vi "GUI_picoscope.vi"() -> ()   [LabVIEW 2020]
uses:
  Device Drivers/ScopeAnalysis/SubVis/method_TypDef.ctl
  Device Drivers/ScopeAnalysis/SubVis/channels_TypDef.ctl
  Shared/GUI_Template/GUI_master/tcp new data cluster.ctl
  General-Controler/firstCall_TypDef.ctl
panel:
  in  "TimeAxis.Max Sample Points::1":T1(ring)=enum."5k" caption="Max record length"
  in  "Trigger.Source::1":u16(ring) caption="Source" items=["Channel 1", "Channel 2", "Channel 3", "Channel 4", "External", "Power Line"]
  in  "Analysis":T4={"Channel::1"=enum."Analysis1", "Calculations.Method::1"=enum."trigger", "Measurements::1"=-5e-07, "Calculations.Linked::1"=enum."na", "Calculations.Additional::1"=0.0} {"Calculations.Additional::1" min=0.0 max=0.0; "Measurements::1" min=0.0 max=0.0}
  in  "TimeAxis.Time base::1":dbl=500000000.0 caption="Time interval" min=0.0 max=0.0 step=1000000.0 format="%.0p"
  in  "Trigger.mode::1":u16(ring) caption="Mode" items=["Auto", "Normal", "Single", "Single auto trigger"]
  in  "Trigger.Level::1":dbl=0.5 caption="Level" min=0.0 max=0.0 format="%#_6p"
  in  "Trigger.Slope::1":u16(ring) caption="Slope" items=["Rising", "Falling"]
  in  "autoscale::1":bool caption="auto\nscale"
  in  "LocalSavingPath::1":path
  in  "save::1":bool=TRUE caption="save"
  in  "Select device":string(combo)="StagingPXIFast1"
  in  "Refresh Button":bool
  out "device status::1":string="Initialized" caption="Device status"
  in  "stop":bool=TRUE
  out "GUIdevice 1":string="StagingPXIFast1"
  in  "Waveform cluster":T5={"Channel::1"=enum."Channel0", "coupling::1"=1, "Verticaloffset::1"=0.0, "Chenabled::1"=1, "verticalrange::1"=0.1, "Names::1"="", "scopeTraceGUI::1"=[{"t0"=timestamp(-4.999999999588667e-07 s since 1904-01-01), "dt"=2e-09, "Y"=array[1000 elements]}, {"t0"=timestamp(-4.999999999588667e-07 s since 1904-01-01), "dt"=2e-09, "Y"=array[1000 elements]}]} {"verticalrange::1" min=0.0001 max=30.0 format="%_4f"; "Chenabled::1" items=["off", "on"]; "Verticaloffset::1" min=-5.0 max=5.0; "coupling::1" items=["AC", "DC"]}
  # "TRIGGER"
  # "HORIZONTAL"
  # "ANALYSIS"
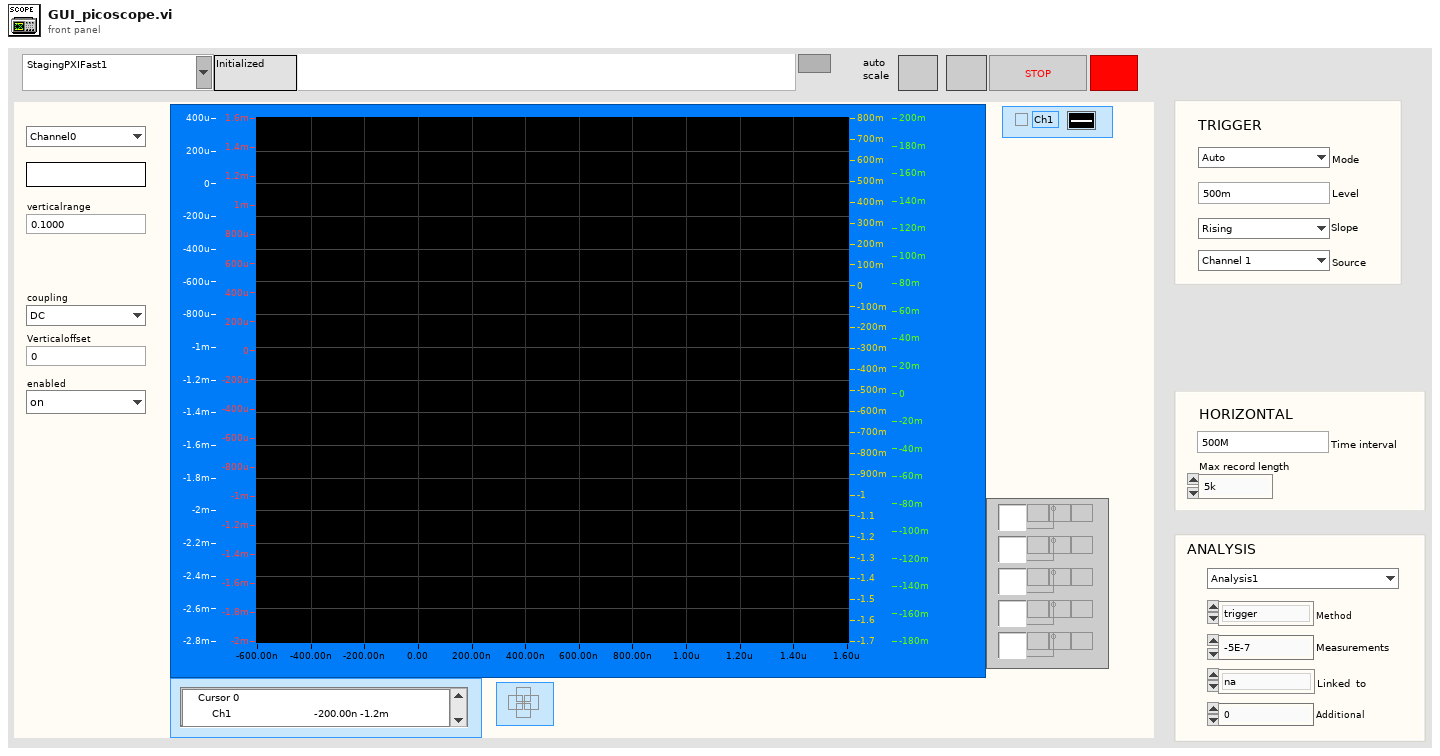
[diagram p1: front panel]
types:
  T1 = enum16{"50", "100", "250", "500", "1000", "2500", "5k", "10k", "25k", "50k", "100k", "250k", "500k", "1M", "2M", "2.5M", "5M", "10M", "25M", "50M", "100M"}
  T2 = typedef "method_TypDef.ctl" = enum16{"n/a", "max", "min", "energy", "trigger", "maxtime", "mintime"}
  T3 = typedef "channels_TypDef.ctl" = enum16{"na", "StagingPXIFast1 scopeTrace.Channel0", "StagingPXIFast1 scopeTrace.Channel1", "StagingPXIFast2 scopeTrace.Channel0", "StagingPXIFast2 scopeTrace.Channel1", "StagingPXISlow scopeTrace.Channel0", "StagingPXISlow scopeTrace.Channel1", "StagingPXISlow scopeTrace.Channel2", "StagingPXISlow scopeTrace.Channel3", "StagingPXISlow scopeTrace.Channel4", "StagingPXISlow scopeTrace.Channel5", "StagingPXISlow scopeTrace.Channel6", "StagingPXISlow scopeTrace.Channel7"}
  T4 = cluster{"Channel::1":enum16{"Analysis1", "Analysis2", "Analysis3", "Analysis4", "Analysis5", "Analysis6", "Analysis7", "Analysis8", "Analysis9"}, "Calculations.Method::1":T2, "Measurements::1":dbl, "Calculations.Linked::1":T3, "Calculations.Additional::1":dbl}
  T5 = cluster{"Channel::1":enum16{"Channel0", "Channel1", "Channel2", "Channel3", "Channel4", "Channel5", "Channel6", "Channel7"}, "coupling::1":u16, "Verticaloffset::1":dbl, "Chenabled::1":u16, "verticalrange::1":dbl, "Names::1":string, "scopeTraceGUI::1":waveform(dbl)[]}
  T6 = typedef "tcp new data cluster.ctl" = cluster{"EventEnum":enum16{"new data", "connection status update"}, "Device name":string}
  T7 = typedef "firstCall_TypDef.ctl" = enum16{"reset", "read"}
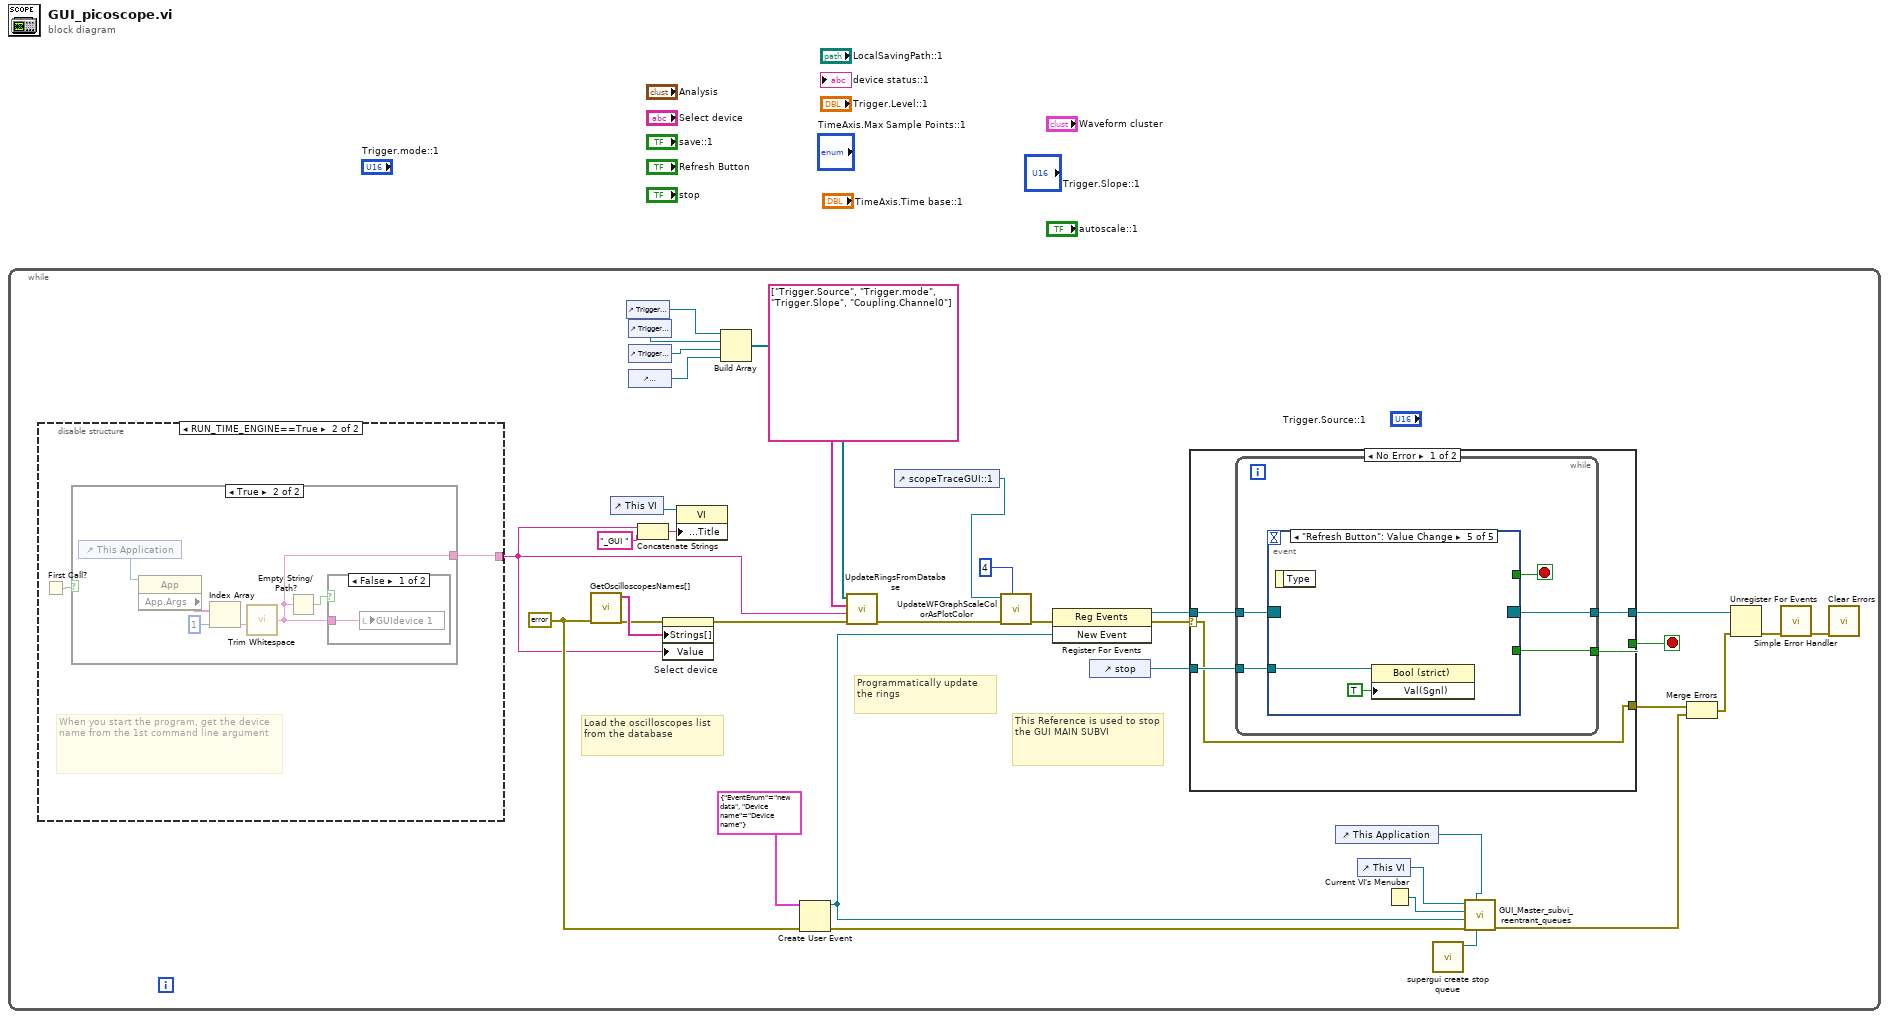
[diagram p0: block diagram]
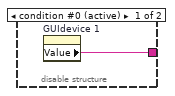
[diagram p2: hidden frame]
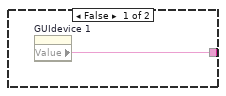
[diagram p3: hidden frame]
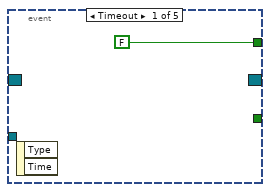
[diagram p5: hidden frame]
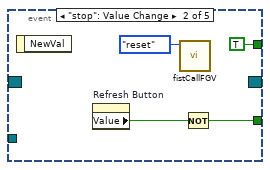
[diagram p6: hidden frame]
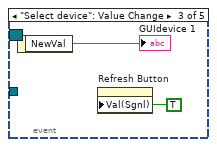
[diagram p7: hidden frame]
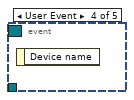
[diagram p8: hidden frame]
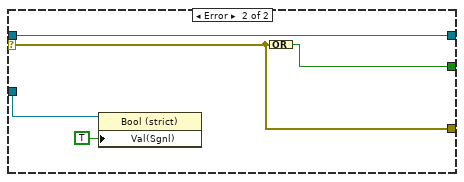
[diagram p9: hidden frame]
diagram:
  n1 = while {
    stop <- w33 stop-if-true
    w7 = errorcluster {"status"=FALSE, "code"=0, "source"=""} ("error in (no error)")
    # "Programmatically update the rings"
    # "Load the oscilloscopes list from the database"
    # "This Reference is used to stop the GUI MAIN SUBVI"
    n2 = disable-structure shown="RUN_TIME_ENGINE==True" {
      disable-tunnel: [w36 w37] -> w1
      frame condition #0 (active) {
        n3 = property on="GUIdevice 1" class="Str"() -> ("Value"=w36:string)  [unwired: 2 in, 2 out]
      }
      frame condition #1 {
        # "When you start the program, get the device name from the 1st command line argument"
        n4 = First Call?() -> (First Call?: T/F=w38:bool)
        n5 = case shown="True" w38 {
          tunnel: [w39 w40] -> w37
          frame False {
            n6 = property on="GUIdevice 1" class="Str"() -> ("Value"=w39:string)  [unwired: 2 in, 2 out]
          }
          frame True {
            n7 = control-ref of="This Application"() -> (w42:refnum<vi>)
            n8 = property class="App"(reference=w42) -> ("App.Args"=w43:string[])  [unwired: 1 in, 2 out]
            n9 = Index Array(array=w43, index=1) -> (element=w44:string)
            n10 = call <vilib>:"Trim Whitespace.vi"("string"=w44) -> ("trimmed string"=w40:string)  [unwired: 1 in]
            n11 = Empty String/Path?(string/path=w40) -> (empty?=w45:bool)
            n12 = case shown="False" w45 {
              tunnel: w40 -> [w46 _]
              frame False {
                n13 = local write "GUIdevice 1"(w46) -> ()
              }
              frame True {
              }
            }
          }
        }
      }
    }
    n14 = call "GetOscilloscopesNames[].vi"("error in (no error)"=w7) -> ("error IO"=w24:errorcluster, "OscilloscopesNames[]"=w25:string[])  [unwired: 9 in]
    n15 = control-ref of="This VI"() -> (w4:refnum<vi>)
    n16 = control-ref of="Trigger.Source::1"() -> (w6:refnum<vi>)
    n17 = control-ref of="Trigger.mode::1"() -> (w22:refnum<vi>)
    n18 = control-ref of="Trigger.Slope::1"() -> (w21:refnum<vi>)
    n19 = control-ref of="Coupling::1"() -> (w20:refnum<vi>)
    n20 = Concatenate Strings(w1, "_GUI ") -> (w3:string)
    n21 = property on="Select device" class="CmbBox"(error in=w24, "Strings[]"=w25, "Value"=w1) -> (error out=w23:errorcluster)  [unwired: 1 in, 1 out]
    n22 = property class="VI"(reference=w4, "Front Panel.Title"=w3) -> ()  [unwired: 1 in, 2 out]
    n23 = Build Array(w6, w22, w21, w20) -> (w19:refnum<vi>[])
    n24 = Create User Event(user event datatype=T6 {"EventEnum"=enum."new data", "Device name"="Device name"} ("New Event"), error in=w7) -> (user event=w27:refnum<user-event>, error out=w28:errorcluster)
    n25 = call "UpdateRingsFromDatabase.vi"("error in (no error)"=w23, "device"=w1, "VariablesNames[]"=string[] ["Trigger.Source", "Trigger.mode", "Trigger.Slope", "Coupling.Channel0"], "RingsRefs[]"=w19) -> ("error out"=w16:errorcluster)  [unwired: 7 in]
    n26 = control-ref of="scopeTraceGUI::1"() -> (w10:refnum<vi>)
    n27 = call "UpdateWFGraphScaleColorAsPlotColor.vi"("Plots#"=4, "error in (no error)"=w16, "WaveformGraph in"=w10) -> ("error out"=w15:errorcluster)  [unwired: 8 in]
    n28 = register-events(error in=w15, w27) -> (reference out=w35:refnum<event-registration>, error out=w14:errorcluster)  [unwired: 1 in]
    n29 = control-ref of="stop"() -> (w32:refnum<vi>)
    n30 = case shown="No Error" w14 {
      selector: w14 -> [w47 w66]
      tunnel: w35 -> [w51 w68]
      tunnel: [w50 w68] -> w34
      tunnel: [w49 w67] -> w33
      tunnel: w32 -> [w48 w69]
      tunnel: [w47 w66] -> w12
      frame No Error {
        n31 = while {
          tunnel: w51 -> [w56]
          tunnel: [w55] -> w50
          tunnel: [w53] -> w49
          tunnel: w48 -> [w52]
          stop <- w54 stop-if-true
          n32 = event shown="[4] \"Refresh Button\": Value Change" {
            selector: w56 -> [_ _ _ _ _]
            dyn-events: [_ _ _ _ _] -> w55
            timeout: _ -> [_ _ _ _ _]
            tunnel: [FALSE TRUE _ _ _] -> w54
            tunnel: [_ w59 _ _ _] -> w53
            tunnel: w52 -> [_ _ _ _ w65]
            event Timeout {
              n33 = event-data() -> ()  [unwired: 1 in, 2 out]
            }
            event "stop": Value Change {
              n34 = event-data() -> ()  [unwired: 1 in, 1 out]
              n35 = property on="Refresh Button" class="Bool (strict)"() -> ("Value"=w60:bool)  [unwired: 2 in, 2 out]
              n36 = call "fistCallFGV.vi"("Function"=firstCall_TypDef."reset") -> ()  [unwired: 9 in, 2 out]
              n37 = Not(x=w60) -> (.not. x?=w59:bool)
            }
            event "Select device": Value Change {
              n38 = event-data() -> ("NewVal"=→"GUIdevice 1":string)  [unwired: 1 in]
              n39 = property on="Refresh Button" class="Bool (strict)"("Val(Sgnl)"=TRUE ("Value (Signaling)")) -> ()  [unwired: 2 in, 2 out]
            }
            event User Event {
              n40 = event-data() -> ()  [unwired: 1 in, 1 out]
            }
            event "Refresh Button": Value Change {
              n41 = event-data() -> ()  [unwired: 1 in, 1 out]
              n42 = property class="Bool (strict)"(reference=w65, "Val(Sgnl)"=TRUE ("Value (Signaling)")) -> ()  [unwired: 1 in, 2 out]
            }
          }
        }
      }
      frame Error {
        n43 = property class="Bool (strict)"(reference=w69, "Val(Sgnl)"=TRUE ("Value (Signaling)")) -> ()  [unwired: 1 in, 2 out]
        n44 = Compound Arithmetic op=OR(w66) -> (w67:bool)
      }
    }
    n45 = control-ref of="This Application"() -> (w26:refnum<vi>)
    n46 = control-ref of="This VI"() -> (w31:refnum<vi>)
    n47 = Current VI's Menubar() -> (w30:refnum<k9>)
    n48 = call "supergui create stop queue.vi"() -> ("STOP Queue out"=w5:refnum<queue>)  [unwired: 11 in]
    n49 = call "GUI_Master_subvi_reentrant_queues.vi"("STOP Queue in"=w5, "This Application"=w26, "error in (no error)"=w28, "tcp data event"=w27, "Caller menu reference"=w30, "Caller VI ref"=w31) -> ("error out"=w13:errorcluster)  [unwired: 5 in]
    n50 = Merge Errors(w12, w13) -> (w11:errorcluster)
    n51 = Unregister For Events(event registration refnum=w34, error in=w11) -> (error out=w9:errorcluster)
    n52 = call <vilib>:"Simple Error Handler.vi"("error in (no error)"=w9) -> ("error out"=w8:errorcluster)  [unwired: 4 in, 4 out]
    n53 = call <vilib>:"Clear Errors.vi"("error in (no error)"=w8) -> ()  [unwired: 5 in, 2 out]
  }
